vi "Punto 3.vi"() -> ()   [LabVIEW 2020]
panel:
  in  "Stop buttom":bool
  out "Value of destiny scale":dbl
  in  "Value of original scale":dbl
  in  "Operate":bool
  in  "Destiny scale":string(combo)
  in  "Original scale":string(combo)
  # "This program was created by Juan Bermúdez from the Army Aviation School\nat the Aircraft Engineering of the assignature of Programation II"
  # "How to use the software?:\n1- First, select the scale of longitude original.\n2- Second, select the new scale of longitude.\n3- Third, write the value of the longitude.\n4- Forth, push the buttom called = ''Operate''.\n5- Fifth, if you want to stop the software, push the buttom called = ''Stop buttom''.\n Enjoy the software :)"
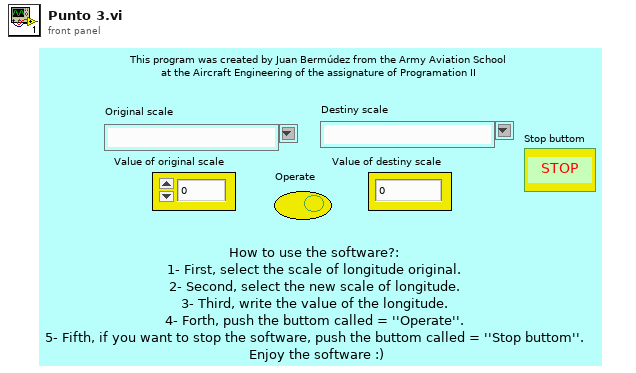
[diagram p1: front panel]
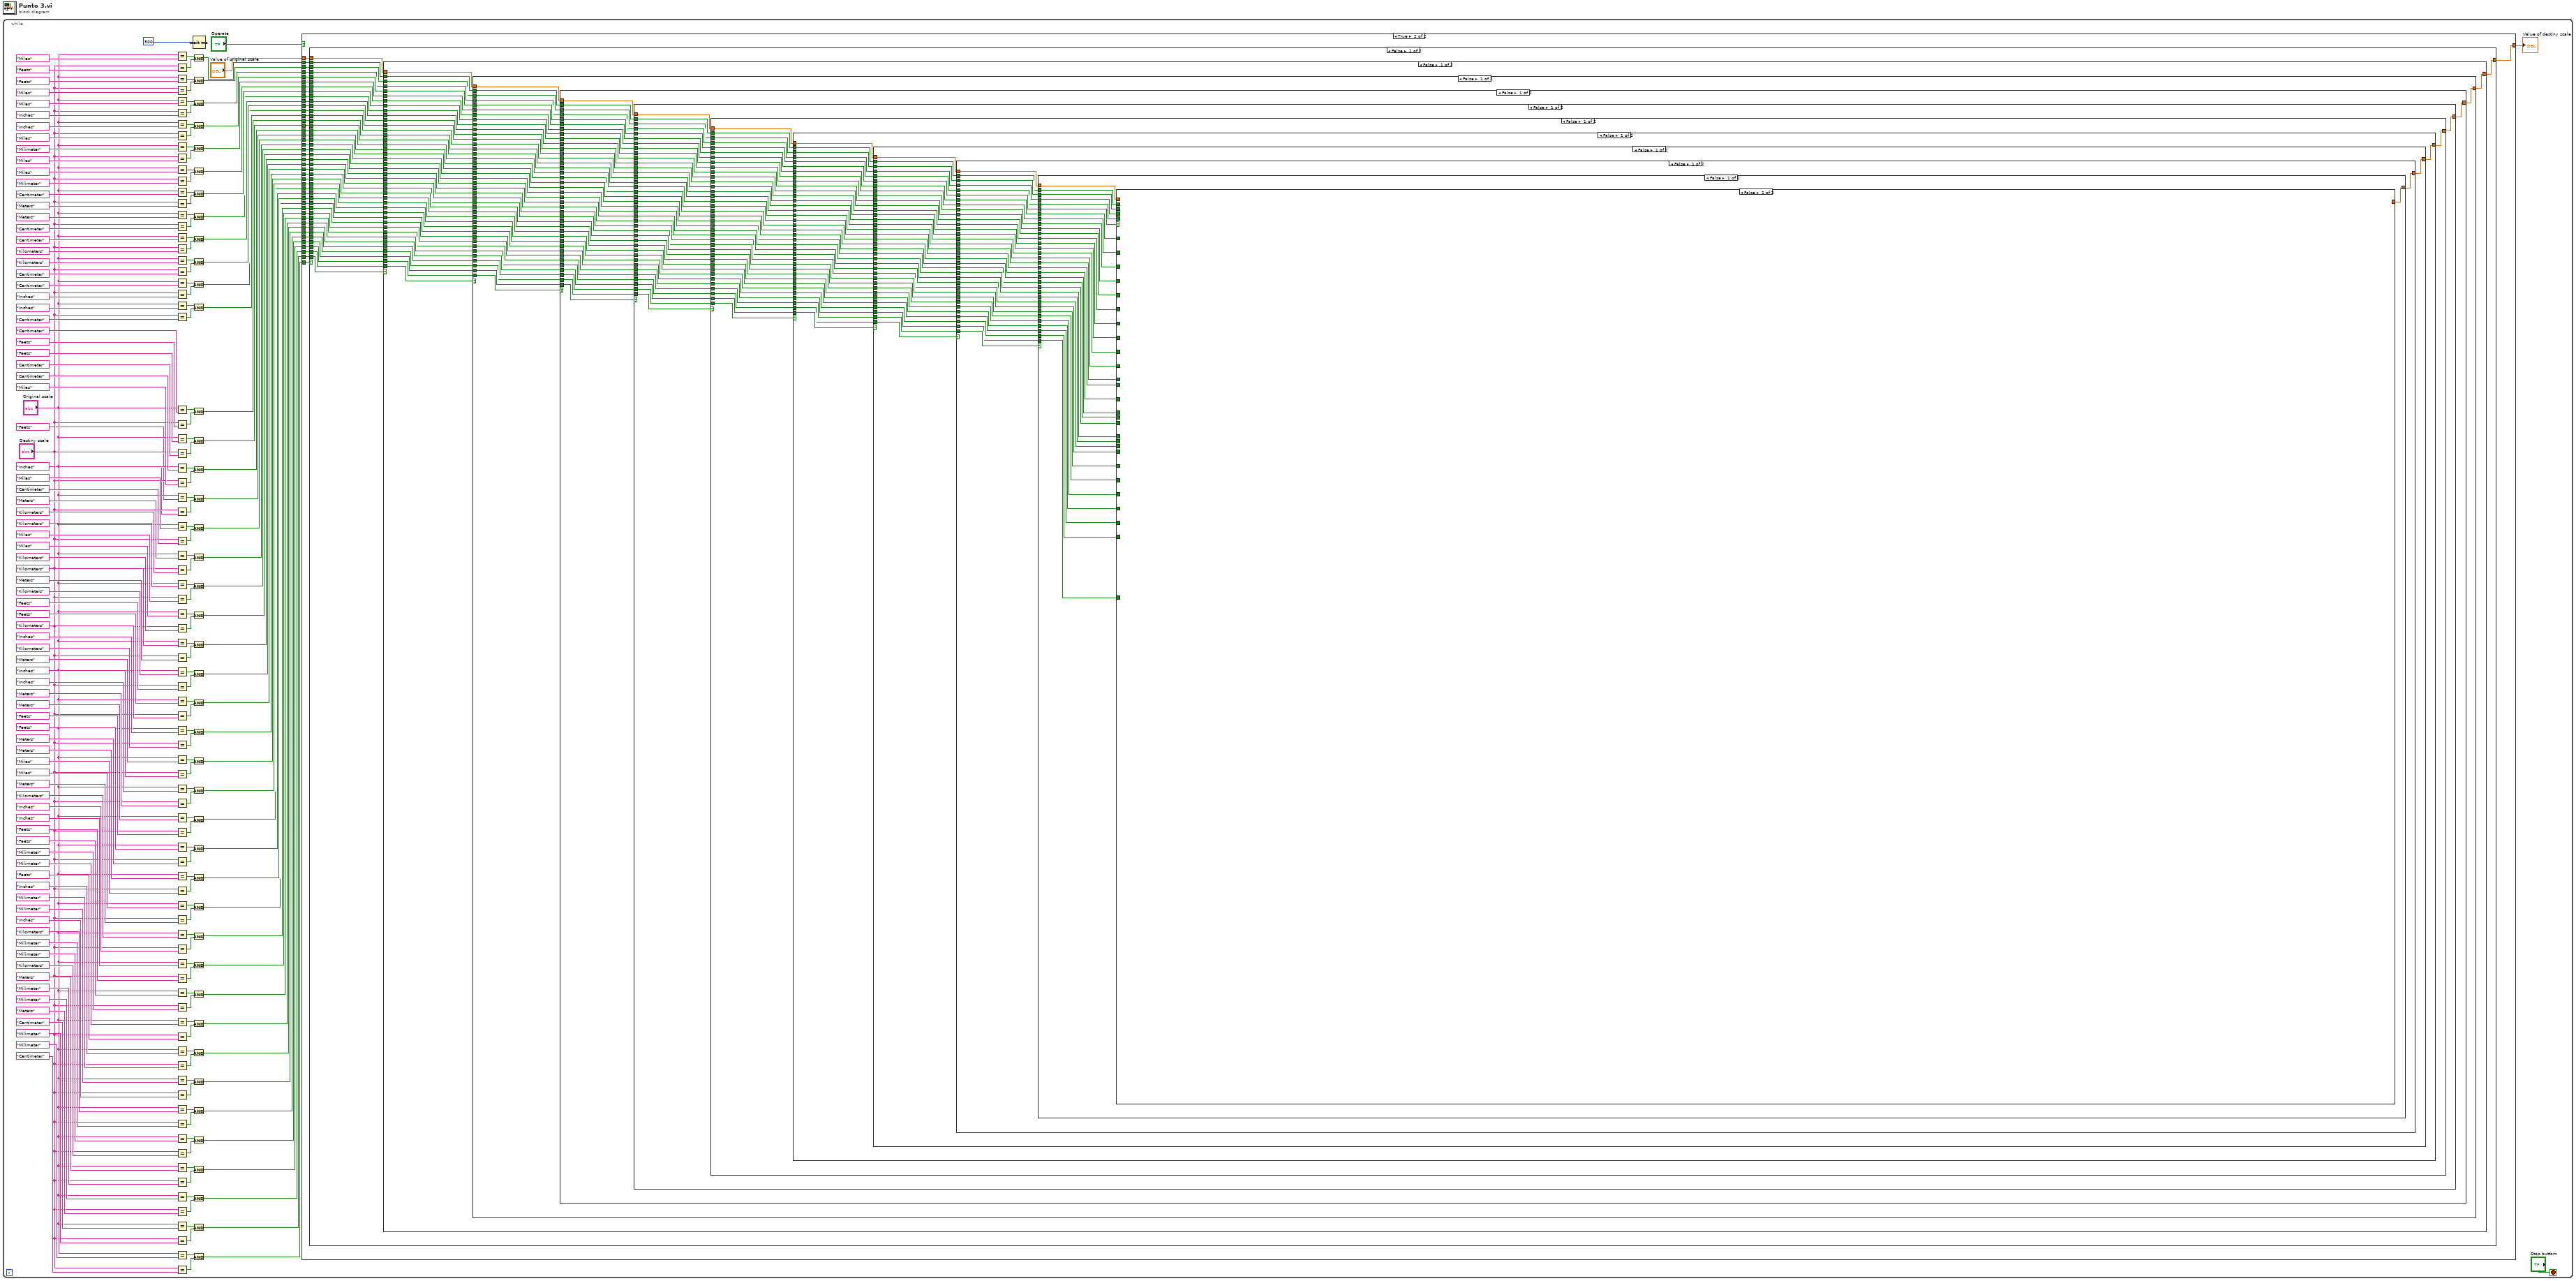
[diagram p0: block diagram]
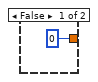
[diagram p2: hidden frame]
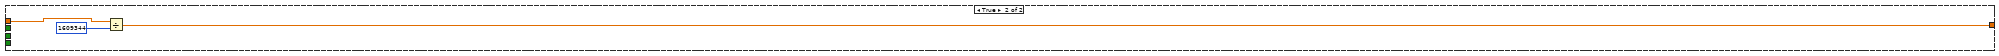
[diagram p3: hidden frame]
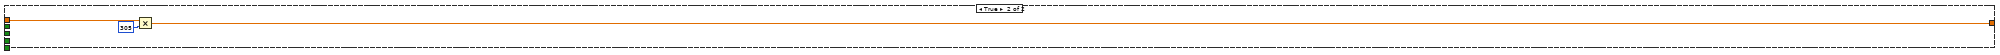
[diagram p4: hidden frame]
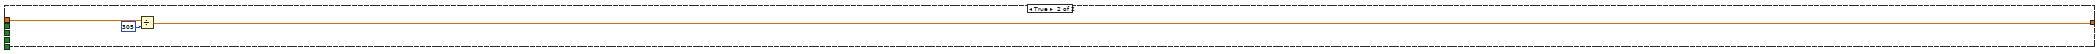
[diagram p5: hidden frame]
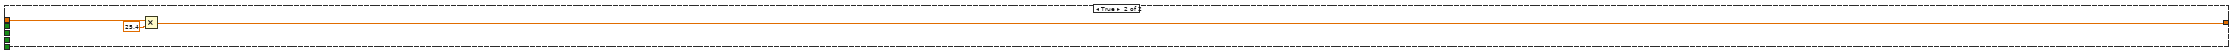
[diagram p6: hidden frame]
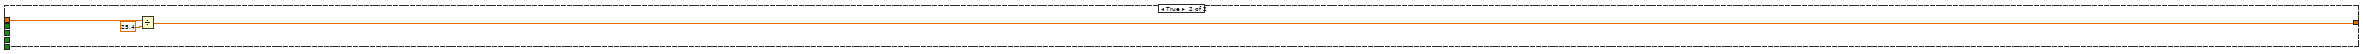
[diagram p7: hidden frame]
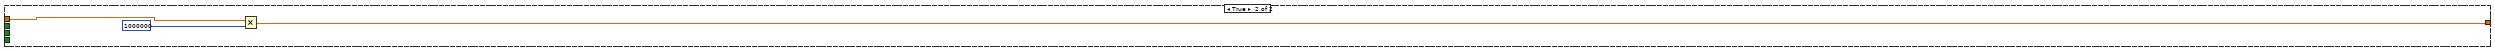
[diagram p8: hidden frame]
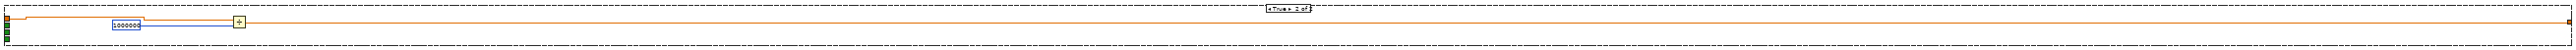
[diagram p9: hidden frame]
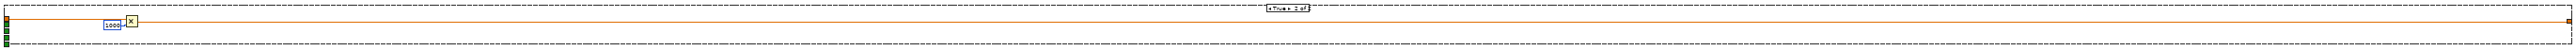
[diagram p10: hidden frame]
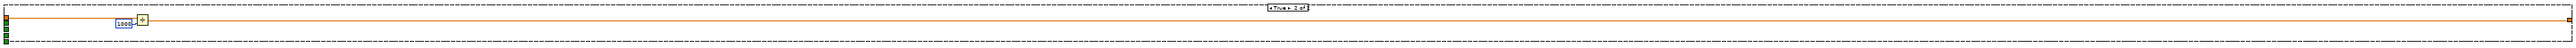
[diagram p11: hidden frame]
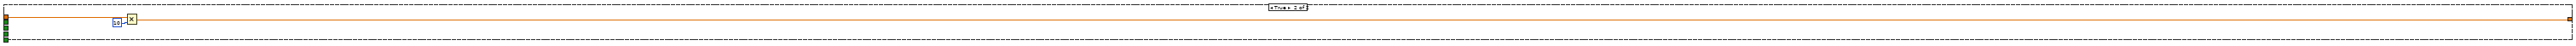
[diagram p12: hidden frame]
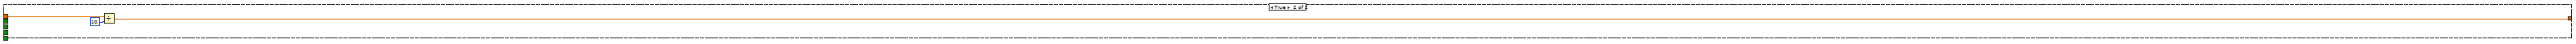
[diagram p13: hidden frame]
diagram:
  n1 = while {
    stop <- "Stop buttom" stop-if-true
    n2 = Equal?(x="Original scale", y="Miles") -> (x = y?=w10:bool)
    n3 = Equal?(x="Destiny scale", y="Feets") -> (x = y?=w11:bool)
    n4 = Equal?(x="Original scale", y="Feets") -> (x = y?=w16:bool)
    n5 = Equal?(x="Destiny scale", y="Miles") -> (x = y?=w15:bool)
    n6 = Equal?(x="Original scale", y="Miles") -> (x = y?=w20:bool)
    n7 = Equal?(x="Destiny scale", y="Inches") -> (x = y?=w21:bool)
    n8 = Equal?(x="Original scale", y="Inches") -> (x = y?=w26:bool)
    n9 = Equal?(x="Destiny scale", y="Miles") -> (x = y?=w25:bool)
    n10 = Equal?(x="Original scale", y="Milimeter") -> (x = y?=w163:bool)
    n11 = Equal?(x="Destiny scale", y="Miles") -> (x = y?=w164:bool)
    n12 = Equal?(x="Original scale", y="Miles") -> (x = y?=w159:bool)
    n13 = Equal?(x="Destiny scale", y="Milimeter") -> (x = y?=w158:bool)
    n14 = Equal?(x="Original scale", y="Centimeter") -> (x = y?=w153:bool)
    n15 = Equal?(x="Destiny scale", y="Meters") -> (x = y?=w154:bool)
    n16 = Equal?(x="Original scale", y="Meters") -> (x = y?=w148:bool)
    n17 = Equal?(x="Destiny scale", y="Centimeter") -> (x = y?=w149:bool)
    n18 = Equal?(x="Original scale", y="Centimeter") -> (x = y?=w143:bool)
    n19 = Equal?(x="Destiny scale", y="Kilometers") -> (x = y?=w144:bool)
    n20 = Equal?(x="Original scale", y="Kilometers") -> (x = y?=w139:bool)
    n21 = Equal?(x="Destiny scale", y="Centimeter") -> (x = y?=w138:bool)
    n22 = Equal?(x="Original scale", y="Centimeter") -> (x = y?=w133:bool)
    n23 = Equal?(x="Destiny scale", y="Inches") -> (x = y?=w134:bool)
    n24 = Equal?(x="Original scale", y="Inches") -> (x = y?=w128:bool)
    n25 = Equal?(x="Destiny scale", y="Centimeter") -> (x = y?=w129:bool)
    n26 = Equal?(x="Original scale", y="Centimeter") -> (x = y?=w123:bool)
    n27 = Equal?(x="Destiny scale", y="Feets") -> (x = y?=w124:bool)
    n28 = Equal?(x="Original scale", y="Feets") -> (x = y?=w118:bool)
    n29 = Equal?(x="Destiny scale", y="Centimeter") -> (x = y?=w119:bool)
    n30 = Equal?(x="Original scale", y="Centimeter") -> (x = y?=w114:bool)
    n31 = Equal?(x="Destiny scale", y="Miles") -> (x = y?=w113:bool)
    n32 = Equal?(x="Original scale", y="Feets") -> (x = y?=w32:bool)
    n33 = Equal?(x="Destiny scale", y="Inches") -> (x = y?=w31:bool)
    n34 = Equal?(x="Original scale", y="Miles") -> (x = y?=w108:bool)
    n35 = Equal?(x="Destiny scale", y="Centimeter") -> (x = y?=w109:bool)
    n36 = Equal?(x="Original scale", y="Meters") -> (x = y?=w103:bool)
    n37 = Equal?(x="Destiny scale", y="Kilometers") -> (x = y?=w104:bool)
    n38 = Equal?(x="Original scale", y="Kilometers") -> (x = y?=w41:bool)
    n39 = Equal?(x="Destiny scale", y="Miles") -> (x = y?=w42:bool)
    n40 = Equal?(x="Original scale", y="Miles") -> (x = y?=w44:bool)
    n41 = Equal?(x="Destiny scale", y="Kilometers") -> (x = y?=w43:bool)
    n42 = Equal?(x="Original scale", y="Kilometers") -> (x = y?=w98:bool)
    n43 = Equal?(x="Destiny scale", y="Meters") -> (x = y?=w99:bool)
    n44 = Equal?(x="Original scale", y="Kilometers") -> (x = y?=w54:bool)
    n45 = Equal?(x="Destiny scale", y="Feets") -> (x = y?=w53:bool)
    n46 = Equal?(x="Original scale", y="Feets") -> (x = y?=w48:bool)
    n47 = Equal?(x="Destiny scale", y="Kilometers") -> (x = y?=w49:bool)
    n48 = Equal?(x="Original scale", y="Inches") -> (x = y?=w59:bool)
    n49 = Equal?(x="Destiny scale", y="Kilometers") -> (x = y?=w58:bool)
    n50 = Equal?(x="Original scale", y="Meters") -> (x = y?=w93:bool)
    n51 = Equal?(x="Destiny scale", y="Inches") -> (x = y?=w94:bool)
    n52 = Equal?(x="Original scale", y="Inches") -> (x = y?=w89:bool)
    n53 = Equal?(x="Destiny scale", y="Meters") -> (x = y?=w88:bool)
    n54 = Equal?(x="Original scale", y="Meters") -> (x = y?=w83:bool)
    n55 = Equal?(x="Destiny scale", y="Feets") -> (x = y?=w84:bool)
    n56 = Equal?(x="Original scale", y="Feets") -> (x = y?=w82:bool)
    n57 = Equal?(x="Destiny scale", y="Meters") -> (x = y?=w81:bool)
    n58 = Equal?(x="Original scale", y="Meters") -> (x = y?=w74:bool)
    n59 = Equal?(x="Destiny scale", y="Miles") -> (x = y?=w73:bool)
    n60 = Equal?(x="Original scale", y="Miles") -> (x = y?=w71:bool)
    n61 = Equal?(x="Destiny scale", y="Meters") -> (x = y?=w72:bool)
    n62 = Equal?(x="Original scale", y="Kilometers") -> (x = y?=w63:bool)
    n63 = Equal?(x="Destiny scale", y="Inches") -> (x = y?=w64:bool)
    n64 = Equal?(x="Original scale", y="Inches") -> (x = y?=w33:bool)
    n65 = Equal?(x="Destiny scale", y="Feets") -> (x = y?=w34:bool)
    n66 = Equal?(x="Original scale", y="Feets") -> (x = y?=w168:bool)
    n67 = Equal?(x="Destiny scale", y="Milimeter") -> (x = y?=w169:bool)
    n68 = Equal?(x="Original scale", y="Milimeter") -> (x = y?=w174:bool)
    n69 = Equal?(x="Destiny scale", y="Feets") -> (x = y?=w173:bool)
    n70 = Equal?(x="Original scale", y="Inches") -> (x = y?=w179:bool)
    n71 = Equal?(x="Destiny scale", y="Milimeter") -> (x = y?=w178:bool)
    n72 = Equal?(x="Original scale", y="Milimeter") -> (x = y?=w183:bool)
    n73 = Equal?(x="Destiny scale", y="Inches") -> (x = y?=w184:bool)
    n74 = Equal?(x="Original scale", y="Kilometers") -> (x = y?=w188:bool)
    n75 = Equal?(x="Destiny scale", y="Milimeter") -> (x = y?=w189:bool)
    n76 = Equal?(x="Original scale", y="Milimeter") -> (x = y?=w194:bool)
    n77 = Equal?(x="Destiny scale", y="Kilometers") -> (x = y?=w193:bool)
    n78 = Equal?(x="Original scale", y="Meters") -> (x = y?=w198:bool)
    n79 = Equal?(x="Destiny scale", y="Milimeter") -> (x = y?=w199:bool)
    n80 = Equal?(x="Original scale", y="Milimeter") -> (x = y?=w204:bool)
    n81 = Equal?(x="Destiny scale", y="Meters") -> (x = y?=w203:bool)
    n82 = Equal?(x="Original scale", y="Centimeter") -> (x = y?=w208:bool)
    n83 = Equal?(x="Destiny scale", y="Milimeter") -> (x = y?=w209:bool)
    n84 = Equal?(x="Original scale", y="Milimeter") -> (x = y?=w215:bool)
    n85 = Equal?(x="Destiny scale", y="Centimeter") -> (x = y?=w214:bool)
    n86 = And(x=w10, y=w11) -> (x .and. y?=w5:bool)
    n87 = And(x=w16, y=w15) -> (x .and. y?=w12:bool)
    n88 = And(x=w20, y=w21) -> (x .and. y?=w17:bool)
    n89 = And(x=w26, y=w25) -> (x .and. y?=w22:bool)
    n90 = And(x=w163, y=w164) -> (x .and. y?=w160:bool)
    n91 = And(x=w159, y=w158) -> (x .and. y?=w155:bool)
    n92 = And(x=w153, y=w154) -> (x .and. y?=w150:bool)
    n93 = And(x=w148, y=w149) -> (x .and. y?=w145:bool)
    n94 = And(x=w143, y=w144) -> (x .and. y?=w140:bool)
    n95 = And(x=w139, y=w138) -> (x .and. y?=w137:bool)
    n96 = And(x=w133, y=w134) -> (x .and. y?=w130:bool)
    n97 = And(x=w128, y=w129) -> (x .and. y?=w125:bool)
    n98 = And(x=w123, y=w124) -> (x .and. y?=w120:bool)
    n99 = And(x=w118, y=w119) -> (x .and. y?=w115:bool)
    n100 = And(x=w114, y=w113) -> (x .and. y?=w110:bool)
    n101 = And(x=w32, y=w31) -> (x .and. y?=w27:bool)
    n102 = And(x=w108, y=w109) -> (x .and. y?=w105:bool)
    n103 = And(x=w103, y=w104) -> (x .and. y?=w100:bool)
    n104 = And(x=w41, y=w42) -> (x .and. y?=w38:bool)
    n105 = And(x=w44, y=w43) -> (x .and. y?=w35:bool)
    n106 = And(x=w98, y=w99) -> (x .and. y?=w95:bool)
    n107 = And(x=w54, y=w53) -> (x .and. y?=w50:bool)
    n108 = And(x=w48, y=w49) -> (x .and. y?=w45:bool)
    n109 = And(x=w59, y=w58) -> (x .and. y?=w55:bool)
    n110 = And(x=w93, y=w94) -> (x .and. y?=w90:bool)
    n111 = And(x=w89, y=w88) -> (x .and. y?=w85:bool)
    n112 = And(x=w83, y=w84) -> (x .and. y?=w78:bool)
    n113 = And(x=w82, y=w81) -> (x .and. y?=w75:bool)
    n114 = And(x=w74, y=w73) -> (x .and. y?=w66:bool)
    n115 = And(x=w71, y=w72) -> (x .and. y?=w65:bool)
    n116 = And(x=w63, y=w64) -> (x .and. y?=w60:bool)
    n117 = And(x=w33, y=w34) -> (x .and. y?=w28:bool)
    n118 = And(x=w168, y=w169) -> (x .and. y?=w165:bool)
    n119 = And(x=w174, y=w173) -> (x .and. y?=w170:bool)
    n120 = And(x=w179, y=w178) -> (x .and. y?=w175:bool)
    n121 = And(x=w183, y=w184) -> (x .and. y?=w180:bool)
    n122 = And(x=w188, y=w189) -> (x .and. y?=w185:bool)
    n123 = And(x=w194, y=w193) -> (x .and. y?=w190:bool)
    n124 = And(x=w198, y=w199) -> (x .and. y?=w195:bool)
    n125 = And(x=w204, y=w203) -> (x .and. y?=w200:bool)
    n126 = And(x=w208, y=w209) -> (x .and. y?=w205:bool)
    n127 = And(x=w215, y=w214) -> (x .and. y?=w212:bool)
    n128 = Wait (ms)(milliseconds to wait=500) -> ()  [unwired: 1 out]
    n129 = case shown="True" "Operate" {
      tunnel: w212 -> [_ w262]
      tunnel: "Value of original scale" -> [_ w261]
      tunnel: [0 w260] -> w210
      tunnel: w205 -> [_ w259]
      tunnel: w200 -> [_ w258]
      tunnel: w195 -> [_ w257]
      tunnel: w190 -> [_ w256]
      tunnel: w185 -> [_ w255]
      tunnel: w180 -> [_ w254]
      tunnel: w175 -> [_ w253]
      tunnel: w170 -> [_ w252]
      tunnel: w165 -> [_ w251]
      tunnel: w160 -> [_ w250]
      tunnel: w155 -> [_ w249]
      tunnel: w150 -> [_ w248]
      tunnel: w145 -> [_ w247]
      tunnel: w140 -> [_ w246]
      tunnel: w137 -> [_ w245]
      tunnel: w130 -> [_ w244]
      tunnel: w125 -> [_ w243]
      tunnel: w120 -> [_ w242]
      tunnel: w115 -> [_ w241]
      tunnel: w110 -> [_ w240]
      tunnel: w105 -> [_ w239]
      tunnel: w100 -> [_ w238]
      tunnel: w95 -> [_ w237]
      tunnel: w90 -> [_ w236]
      tunnel: w85 -> [_ w235]
      tunnel: w78 -> [_ w234]
      tunnel: w75 -> [_ w233]
      tunnel: w66 -> [_ w232]
      tunnel: w65 -> [_ w231]
      tunnel: w60 -> [_ w230]
      tunnel: w55 -> [_ w229]
      tunnel: w50 -> [_ w228]
      tunnel: w45 -> [_ w227]
      tunnel: w38 -> [_ w226]
      tunnel: w35 -> [_ w225]
      tunnel: w28 -> [_ w224]
      tunnel: w27 -> [_ w223]
      tunnel: w22 -> [_ w222]
      tunnel: w17 -> [_ w221]
      tunnel: w12 -> [_ w220]
      tunnel: w5 -> [_ w219]
      frame False {
      }
      frame True {
        n130 = case shown="False" w262 {
          tunnel: w261 -> [w304 w1332]
          tunnel: [w303 w1330] -> w260
          tunnel: w259 -> [w305 _]
          tunnel: w258 -> [w302 _]
          tunnel: w257 -> [w301 _]
          tunnel: w256 -> [w300 _]
          tunnel: w255 -> [w299 _]
          tunnel: w254 -> [w298 _]
          tunnel: w253 -> [w297 _]
          tunnel: w252 -> [w296 _]
          tunnel: w251 -> [w295 _]
          tunnel: w250 -> [w294 _]
          tunnel: w249 -> [w293 _]
          tunnel: w248 -> [w292 _]
          tunnel: w247 -> [w291 _]
          tunnel: w246 -> [w290 _]
          tunnel: w245 -> [w289 _]
          tunnel: w244 -> [w288 _]
          tunnel: w243 -> [w287 _]
          tunnel: w242 -> [w286 _]
          tunnel: w241 -> [w285 _]
          tunnel: w240 -> [w284 _]
          tunnel: w239 -> [w283 _]
          tunnel: w238 -> [w282 _]
          tunnel: w237 -> [w281 _]
          tunnel: w236 -> [w280 _]
          tunnel: w235 -> [w279 _]
          tunnel: w234 -> [w278 _]
          tunnel: w233 -> [w277 _]
          tunnel: w232 -> [w276 _]
          tunnel: w231 -> [w275 _]
          tunnel: w230 -> [w274 _]
          tunnel: w229 -> [w273 _]
          tunnel: w228 -> [w272 _]
          tunnel: w227 -> [w271 _]
          tunnel: w226 -> [w270 _]
          tunnel: w225 -> [w269 _]
          tunnel: w224 -> [w268 _]
          tunnel: w223 -> [w267 _]
          tunnel: w222 -> [w266 _]
          tunnel: w221 -> [w265 _]
          tunnel: w220 -> [w264 _]
          tunnel: w219 -> [w263 _]
          frame False {
            n131 = case shown="False" w305 {
              tunnel: w304 -> [w346 w1329]
              tunnel: [w345 w1327] -> w303
              tunnel: w302 -> [w347 _]
              tunnel: w301 -> [w344 _]
              tunnel: w300 -> [w343 _]
              tunnel: w299 -> [w342 _]
              tunnel: w298 -> [w341 _]
              tunnel: w297 -> [w340 _]
              tunnel: w296 -> [w339 _]
              tunnel: w295 -> [w338 _]
              tunnel: w294 -> [w337 _]
              tunnel: w293 -> [w336 _]
              tunnel: w292 -> [w335 _]
              tunnel: w291 -> [w334 _]
              tunnel: w290 -> [w333 _]
              tunnel: w289 -> [w332 _]
              tunnel: w288 -> [w331 _]
              tunnel: w287 -> [w330 _]
              tunnel: w286 -> [w329 _]
              tunnel: w285 -> [w328 _]
              tunnel: w284 -> [w327 _]
              tunnel: w283 -> [w326 _]
              tunnel: w282 -> [w325 _]
              tunnel: w281 -> [w324 _]
              tunnel: w280 -> [w323 _]
              tunnel: w279 -> [w322 _]
              tunnel: w278 -> [w321 _]
              tunnel: w277 -> [w320 _]
              tunnel: w276 -> [w319 _]
              tunnel: w275 -> [w318 _]
              tunnel: w274 -> [w317 _]
              tunnel: w273 -> [w316 _]
              tunnel: w272 -> [w315 _]
              tunnel: w271 -> [w314 _]
              tunnel: w270 -> [w313 _]
              tunnel: w269 -> [w312 _]
              tunnel: w268 -> [w311 _]
              tunnel: w267 -> [w310 _]
              tunnel: w266 -> [w309 _]
              tunnel: w265 -> [w308 _]
              tunnel: w264 -> [w307 _]
              tunnel: w263 -> [w306 _]
              frame False {
                n132 = case shown="False" w347 {
                  tunnel: w346 -> [w387 w1326]
                  tunnel: [w386 w1324] -> w345
                  tunnel: w344 -> [w388 _]
                  tunnel: w343 -> [w385 _]
                  tunnel: w342 -> [w384 _]
                  tunnel: w341 -> [w383 _]
                  tunnel: w340 -> [w382 _]
                  tunnel: w339 -> [w381 _]
                  tunnel: w338 -> [w380 _]
                  tunnel: w337 -> [w379 _]
                  tunnel: w336 -> [w378 _]
                  tunnel: w335 -> [w377 _]
                  tunnel: w334 -> [w376 _]
                  tunnel: w333 -> [w375 _]
                  tunnel: w332 -> [w374 _]
                  tunnel: w331 -> [w373 _]
                  tunnel: w330 -> [w372 _]
                  tunnel: w329 -> [w371 _]
                  tunnel: w328 -> [w370 _]
                  tunnel: w327 -> [w369 _]
                  tunnel: w326 -> [w368 _]
                  tunnel: w325 -> [w367 _]
                  tunnel: w324 -> [w366 _]
                  tunnel: w323 -> [w365 _]
                  tunnel: w322 -> [w364 _]
                  tunnel: w321 -> [w363 _]
                  tunnel: w320 -> [w362 _]
                  tunnel: w319 -> [w361 _]
                  tunnel: w318 -> [w360 _]
                  tunnel: w317 -> [w359 _]
                  tunnel: w316 -> [w358 _]
                  tunnel: w315 -> [w357 _]
                  tunnel: w314 -> [w356 _]
                  tunnel: w313 -> [w355 _]
                  tunnel: w312 -> [w354 _]
                  tunnel: w311 -> [w353 _]
                  tunnel: w310 -> [w352 _]
                  tunnel: w309 -> [w351 _]
                  tunnel: w308 -> [w350 _]
                  tunnel: w307 -> [w349 _]
                  tunnel: w306 -> [w348 _]
                  frame False {
                    n133 = case shown="False" w388 {
                      tunnel: w387 -> [w427 w1323]
                      tunnel: [w426 w1321] -> w386
                      tunnel: w385 -> [w428 _]
                      tunnel: w384 -> [w425 _]
                      tunnel: w383 -> [w424 _]
                      tunnel: w382 -> [w423 _]
                      tunnel: w381 -> [w422 _]
                      tunnel: w380 -> [w421 _]
                      tunnel: w379 -> [w420 _]
                      tunnel: w378 -> [w419 _]
                      tunnel: w377 -> [w418 _]
                      tunnel: w376 -> [w417 _]
                      tunnel: w375 -> [w416 _]
                      tunnel: w374 -> [w415 _]
                      tunnel: w373 -> [w414 _]
                      tunnel: w372 -> [w413 _]
                      tunnel: w371 -> [w412 _]
                      tunnel: w370 -> [w411 _]
                      tunnel: w369 -> [w410 _]
                      tunnel: w368 -> [w409 _]
                      tunnel: w367 -> [w408 _]
                      tunnel: w366 -> [w407 _]
                      tunnel: w365 -> [w406 _]
                      tunnel: w364 -> [w405 _]
                      tunnel: w363 -> [w404 _]
                      tunnel: w362 -> [w403 _]
                      tunnel: w361 -> [w402 _]
                      tunnel: w360 -> [w401 _]
                      tunnel: w359 -> [w400 _]
                      tunnel: w358 -> [w399 _]
                      tunnel: w357 -> [w398 _]
                      tunnel: w356 -> [w397 _]
                      tunnel: w355 -> [w396 _]
                      tunnel: w354 -> [w395 _]
                      tunnel: w353 -> [w394 _]
                      tunnel: w352 -> [w393 _]
                      tunnel: w351 -> [w392 _]
                      tunnel: w350 -> [w391 _]
                      tunnel: w349 -> [w390 _]
                      tunnel: w348 -> [w389 _]
                      frame False {
                        n134 = case shown="False" w428 {
                          tunnel: w427 -> [w466 w1319]
                          tunnel: [w465 w1318] -> w426
                          tunnel: w425 -> [w467 _]
                          tunnel: w424 -> [w464 _]
                          tunnel: w423 -> [w463 _]
                          tunnel: w422 -> [w462 _]
                          tunnel: w421 -> [w461 _]
                          tunnel: w420 -> [w460 _]
                          tunnel: w419 -> [w459 _]
                          tunnel: w418 -> [w458 _]
                          tunnel: w417 -> [w457 _]
                          tunnel: w416 -> [w456 _]
                          tunnel: w415 -> [w455 _]
                          tunnel: w414 -> [w454 _]
                          tunnel: w413 -> [w453 _]
                          tunnel: w412 -> [w452 _]
                          tunnel: w411 -> [w451 _]
                          tunnel: w410 -> [w450 _]
                          tunnel: w409 -> [w449 _]
                          tunnel: w408 -> [w448 _]
                          tunnel: w407 -> [w447 _]
                          tunnel: w406 -> [w446 _]
                          tunnel: w405 -> [w445 _]
                          tunnel: w404 -> [w444 _]
                          tunnel: w403 -> [w443 _]
                          tunnel: w402 -> [w442 _]
                          tunnel: w401 -> [w441 _]
                          tunnel: w400 -> [w440 _]
                          tunnel: w399 -> [w439 _]
                          tunnel: w398 -> [w438 _]
                          tunnel: w397 -> [w437 _]
                          tunnel: w396 -> [w436 _]
                          tunnel: w395 -> [w435 _]
                          tunnel: w394 -> [w434 _]
                          tunnel: w393 -> [w433 _]
                          tunnel: w392 -> [w432 _]
                          tunnel: w391 -> [w431 _]
                          tunnel: w390 -> [w430 _]
                          tunnel: w389 -> [w429 _]
                          frame False {
                            n135 = case shown="False" w467 {
                              tunnel: w466 -> [w504 w1316]
                              tunnel: [w503 w1315] -> w465
                              tunnel: w464 -> [w505 _]
                              tunnel: w463 -> [w502 _]
                              tunnel: w462 -> [w501 _]
                              tunnel: w461 -> [w500 _]
                              tunnel: w460 -> [w499 _]
                              tunnel: w459 -> [w498 _]
                              tunnel: w458 -> [w497 _]
                              tunnel: w457 -> [w496 _]
                              tunnel: w456 -> [w495 _]
                              tunnel: w455 -> [w494 _]
                              tunnel: w454 -> [w493 _]
                              tunnel: w453 -> [w492 _]
                              tunnel: w452 -> [w491 _]
                              tunnel: w451 -> [w490 _]
                              tunnel: w450 -> [w489 _]
                              tunnel: w449 -> [w488 _]
                              tunnel: w448 -> [w487 _]
                              tunnel: w447 -> [w486 _]
                              tunnel: w446 -> [w485 _]
                              tunnel: w445 -> [w484 _]
                              tunnel: w444 -> [w483 _]
                              tunnel: w443 -> [w482 _]
                              tunnel: w442 -> [w481 _]
                              tunnel: w441 -> [w480 _]
                              tunnel: w440 -> [w479 _]
                              tunnel: w439 -> [w478 _]
                              tunnel: w438 -> [w477 _]
                              tunnel: w437 -> [w476 _]
                              tunnel: w436 -> [w475 _]
                              tunnel: w435 -> [w474 _]
                              tunnel: w434 -> [w473 _]
                              tunnel: w433 -> [w472 _]
                              tunnel: w432 -> [w471 _]
                              tunnel: w431 -> [w470 _]
                              tunnel: w430 -> [w469 _]
                              tunnel: w429 -> [w468 _]
                              frame False {
                                n136 = case shown="False" w505 {
                                tunnel: w504 -> [w541 w1314]
                                tunnel: [w540 w1312] -> w503
                                tunnel: w502 -> [w542 _]
                                tunnel: w501 -> [w539 _]
                                tunnel: w500 -> [w538 _]
                                tunnel: w499 -> [w537 _]
                                tunnel: w498 -> [w536 _]
                                tunnel: w497 -> [w535 _]
                                tunnel: w496 -> [w534 _]
                                tunnel: w495 -> [w533 _]
                                tunnel: w494 -> [w532 _]
                                tunnel: w493 -> [w531 _]
                                tunnel: w492 -> [w530 _]
                                tunnel: w491 -> [w529 _]
                                tunnel: w490 -> [w528 _]
                                tunnel: w489 -> [w527 _]
                                tunnel: w488 -> [w526 _]
                                tunnel: w487 -> [w525 _]
                                tunnel: w486 -> [w524 _]
                                tunnel: w485 -> [w523 _]
                                tunnel: w484 -> [w522 _]
                                tunnel: w483 -> [w521 _]
                                tunnel: w482 -> [w520 _]
                                tunnel: w481 -> [w519 _]
                                tunnel: w480 -> [w518 _]
                                tunnel: w479 -> [w517 _]
                                tunnel: w478 -> [w516 _]
                                tunnel: w477 -> [w515 _]
                                tunnel: w476 -> [w514 _]
                                tunnel: w475 -> [w513 _]
                                tunnel: w474 -> [w512 _]
                                tunnel: w473 -> [w511 _]
                                tunnel: w472 -> [w510 _]
                                tunnel: w471 -> [w509 _]
                                tunnel: w470 -> [w508 _]
                                tunnel: w469 -> [w507 _]
                                tunnel: w468 -> [w506 _]
                                frame False {
                                n137 = case shown="False" w542 {
                                tunnel: w541 -> [w577 w1311]
                                tunnel: [w576 w1309] -> w540
                                tunnel: w539 -> [w578 _]
                                tunnel: w538 -> [w575 _]
                                tunnel: w537 -> [w574 _]
                                tunnel: w536 -> [w573 _]
                                tunnel: w535 -> [w572 _]
                                tunnel: w534 -> [w571 _]
                                tunnel: w533 -> [w570 _]
                                tunnel: w532 -> [w569 _]
                                tunnel: w531 -> [w568 _]
                                tunnel: w530 -> [w567 _]
                                tunnel: w529 -> [w566 _]
                                tunnel: w528 -> [w565 _]
                                tunnel: w527 -> [w564 _]
                                tunnel: w526 -> [w563 _]
                                tunnel: w525 -> [w562 _]
                                tunnel: w524 -> [w561 _]
                                tunnel: w523 -> [w560 _]
                                tunnel: w522 -> [w559 _]
                                tunnel: w521 -> [w558 _]
                                tunnel: w520 -> [w557 _]
                                tunnel: w519 -> [w556 _]
                                tunnel: w518 -> [w555 _]
                                tunnel: w517 -> [w554 _]
                                tunnel: w516 -> [w553 _]
                                tunnel: w515 -> [w552 _]
                                tunnel: w514 -> [w551 _]
                                tunnel: w513 -> [w550 _]
                                tunnel: w512 -> [w549 _]
                                tunnel: w511 -> [w548 _]
                                tunnel: w510 -> [w547 _]
                                tunnel: w509 -> [w546 _]
                                tunnel: w508 -> [w545 _]
                                tunnel: w507 -> [w544 _]
                                tunnel: w506 -> [w543 _]
                                frame False {
                                n138 = case shown="False" w578 {
                                tunnel: w577 -> [w612 w1307]
                                tunnel: [w611 w1306] -> w576
                                tunnel: w575 -> [w613 _]
                                tunnel: w574 -> [w610 _]
                                tunnel: w573 -> [w609 _]
                                tunnel: w572 -> [w608 _]
                                tunnel: w571 -> [w607 _]
                                tunnel: w570 -> [w606 _]
                                tunnel: w569 -> [w605 _]
                                tunnel: w568 -> [w604 _]
                                tunnel: w567 -> [w603 _]
                                tunnel: w566 -> [w602 _]
                                tunnel: w565 -> [w601 _]
                                tunnel: w564 -> [w600 _]
                                tunnel: w563 -> [w599 _]
                                tunnel: w562 -> [w598 _]
                                tunnel: w561 -> [w597 _]
                                tunnel: w560 -> [w596 _]
                                tunnel: w559 -> [w595 _]
                                tunnel: w558 -> [w594 _]
                                tunnel: w557 -> [w593 _]
                                tunnel: w556 -> [w592 _]
                                tunnel: w555 -> [w591 _]
                                tunnel: w554 -> [w590 _]
                                tunnel: w553 -> [w589 _]
                                tunnel: w552 -> [w588 _]
                                tunnel: w551 -> [w587 _]
                                tunnel: w550 -> [w586 _]
                                tunnel: w549 -> [w585 _]
                                tunnel: w548 -> [w584 _]
                                tunnel: w547 -> [w583 _]
                                tunnel: w546 -> [w582 _]
                                tunnel: w545 -> [w581 _]
                                tunnel: w544 -> [w580 _]
                                tunnel: w543 -> [w579 _]
                                frame False {
                                n139 = case shown="False" w613 {
                                tunnel: w612 -> [w647 w1305]
                                tunnel: [w645 w1303] -> w611
                                tunnel: w610 -> [w646 _]
                                tunnel: w609 -> [w644 _]
                                tunnel: w608 -> [w643 _]
                                tunnel: w607 -> [w642 _]
                                tunnel: w606 -> [w641 _]
                                tunnel: w605 -> [w640 _]
                                tunnel: w604 -> [w639 _]
                                tunnel: w603 -> [w638 _]
                                tunnel: w602 -> [w637 _]
                                tunnel: w601 -> [w636 _]
                                tunnel: w600 -> [w635 _]
                                tunnel: w599 -> [w634 _]
                                tunnel: w598 -> [w633 _]
                                tunnel: w597 -> [w632 _]
                                tunnel: w596 -> [w631 _]
                                tunnel: w595 -> [w630 _]
                                tunnel: w594 -> [w629 _]
                                tunnel: w593 -> [w628 _]
                                tunnel: w592 -> [w627 _]
                                tunnel: w591 -> [w626 _]
                                tunnel: w590 -> [w625 _]
                                tunnel: w589 -> [w624 _]
                                tunnel: w588 -> [w623 _]
                                tunnel: w587 -> [w622 _]
                                tunnel: w586 -> [w621 _]
                                tunnel: w585 -> [w620 _]
                                tunnel: w584 -> [w619 _]
                                tunnel: w583 -> [w618 _]
                                tunnel: w582 -> [w617 _]
                                tunnel: w581 -> [w616 _]
                                tunnel: w580 -> [w615 _]
                                tunnel: w579 -> [w614 _]
                                frame False {
                                n140 = case shown="False" w646 {
                                tunnel: w647 -> [w680 w1301]
                                tunnel: [w679 w1300] -> w645
                                tunnel: w644 -> [w678 _]
                                tunnel: w643 -> [w677 _]
                                tunnel: w642 -> [w676 _]
                                tunnel: w641 -> [w675 _]
                                tunnel: w640 -> [w674 _]
                                tunnel: w639 -> [w673 _]
                                tunnel: w638 -> [w672 _]
                                tunnel: w637 -> [w671 _]
                                tunnel: w636 -> [w670 _]
                                tunnel: w635 -> [w669 _]
                                tunnel: w634 -> [w668 _]
                                tunnel: w633 -> [w667 _]
                                tunnel: w632 -> [w666 _]
                                tunnel: w631 -> [w665 _]
                                tunnel: w630 -> [w664 _]
                                tunnel: w629 -> [w663 _]
                                tunnel: w628 -> [w662 _]
                                tunnel: w627 -> [w661 _]
                                tunnel: w626 -> [w660 _]
                                tunnel: w625 -> [w659 _]
                                tunnel: w624 -> [w658 _]
                                tunnel: w623 -> [w657 _]
                                tunnel: w622 -> [w656 _]
                                tunnel: w621 -> [w655 _]
                                tunnel: w620 -> [w654 _]
                                tunnel: w619 -> [w653 _]
                                tunnel: w618 -> [w652 _]
                                tunnel: w617 -> [w651 _]
                                tunnel: w616 -> [w650 _]
                                tunnel: w615 -> [w649 _]
                                tunnel: w614 -> [w648 _]
                                frame False {
                                n141 = case shown="False" w678 {
                                tunnel: w680 -> [w711 w1298]
                                tunnel: [w710 w1297] -> w679
                                tunnel: w677 -> [w712 _]
                                tunnel: w676 -> [w709 _]
                                tunnel: w675 -> [w708 _]
                                tunnel: w674 -> [w707 _]
                                tunnel: w673 -> [w706 _]
                                tunnel: w672 -> [w705 _]
                                tunnel: w671 -> [w704 _]
                                tunnel: w670 -> [w703 _]
                                tunnel: w669 -> [w702 _]
                                tunnel: w668 -> [w701 _]
                                tunnel: w667 -> [w700 _]
                                tunnel: w666 -> [w699 _]
                                tunnel: w665 -> [w698 _]
                                tunnel: w664 -> [w697 _]
                                tunnel: w663 -> [w696 _]
                                tunnel: w662 -> [w695 _]
                                tunnel: w661 -> [w694 _]
                                tunnel: w660 -> [w693 _]
                                tunnel: w659 -> [w692 _]
                                tunnel: w658 -> [w691 _]
                                tunnel: w657 -> [w690 _]
                                tunnel: w656 -> [w689 _]
                                tunnel: w655 -> [w688 _]
                                tunnel: w654 -> [w687 _]
                                tunnel: w653 -> [w686 _]
                                tunnel: w652 -> [w685 _]
                                tunnel: w651 -> [w684 _]
                                tunnel: w650 -> [w683 _]
                                tunnel: w649 -> [w682 _]
                                tunnel: w648 -> [w681 _]
                                frame False {
                                n142 = case shown="False" w712 {
                                tunnel: w711 -> [w742 w1295]
                                tunnel: [w741 w1294] -> w710
                                tunnel: w709 -> [w743 _]
                                tunnel: w708 -> [w740 _]
                                tunnel: w707 -> [w739 _]
                                tunnel: w706 -> [w738 _]
                                tunnel: w705 -> [w737 _]
                                tunnel: w704 -> [w736 _]
                                tunnel: w703 -> [w735 _]
                                tunnel: w702 -> [w734 _]
                                tunnel: w701 -> [w733 _]
                                tunnel: w700 -> [w732 _]
                                tunnel: w699 -> [w731 _]
                                tunnel: w698 -> [w730 _]
                                tunnel: w697 -> [w729 _]
                                tunnel: w696 -> [w728 _]
                                tunnel: w695 -> [w727 _]
                                tunnel: w694 -> [w726 _]
                                tunnel: w693 -> [w725 _]
                                tunnel: w692 -> [w724 _]
                                tunnel: w691 -> [w723 _]
                                tunnel: w690 -> [w722 _]
                                tunnel: w689 -> [w721 _]
                                tunnel: w688 -> [w720 _]
                                tunnel: w687 -> [w719 _]
                                tunnel: w686 -> [w718 _]
                                tunnel: w685 -> [w717 _]
                                tunnel: w684 -> [w716 _]
                                tunnel: w683 -> [w715 _]
                                tunnel: w682 -> [w714 _]
                                tunnel: w681 -> [w713 _]
                                frame False {
                                n143 = case shown="False" w743 {
                                tunnel: w742 -> [w772 w1293]
                                tunnel: [w771 w1291] -> w741
                                tunnel: w740 -> [w773 _]
                                tunnel: w739 -> [w770 _]
                                tunnel: w738 -> [w769 _]
                                tunnel: w737 -> [w768 _]
                                tunnel: w736 -> [w767 _]
                                tunnel: w735 -> [w766 _]
                                tunnel: w734 -> [w765 _]
                                tunnel: w733 -> [w764 _]
                                tunnel: w732 -> [w763 _]
                                tunnel: w731 -> [w762 _]
                                tunnel: w730 -> [w761 _]
                                tunnel: w729 -> [w760 _]
                                tunnel: w728 -> [w759 _]
                                tunnel: w727 -> [w758 _]
                                tunnel: w726 -> [w757 _]
                                tunnel: w725 -> [w756 _]
                                tunnel: w724 -> [w755 _]
                                tunnel: w723 -> [w754 _]
                                tunnel: w722 -> [w753 _]
                                tunnel: w721 -> [w752 _]
                                tunnel: w720 -> [w751 _]
                                tunnel: w719 -> [w750 _]
                                tunnel: w718 -> [w749 _]
                                tunnel: w717 -> [w748 _]
                                tunnel: w716 -> [w747 _]
                                tunnel: w715 -> [w746 _]
                                tunnel: w714 -> [w745 _]
                                tunnel: w713 -> [w744 _]
                                frame False {
                                n144 = case shown="False" w773 {
                                tunnel: w772 -> [w801 w1289]
                                tunnel: [w800 w1288] -> w771
                                tunnel: w770 -> [w802 _]
                                tunnel: w769 -> [w799 _]
                                tunnel: w768 -> [w798 _]
                                tunnel: w767 -> [w797 _]
                                tunnel: w766 -> [w796 _]
                                tunnel: w765 -> [w795 _]
                                tunnel: w764 -> [w794 _]
                                tunnel: w763 -> [w793 _]
                                tunnel: w762 -> [w792 _]
                                tunnel: w761 -> [w791 _]
                                tunnel: w760 -> [w790 _]
                                tunnel: w759 -> [w789 _]
                                tunnel: w758 -> [w788 _]
                                tunnel: w757 -> [w787 _]
                                tunnel: w756 -> [w786 _]
                                tunnel: w755 -> [w785 _]
                                tunnel: w754 -> [w784 _]
                                tunnel: w753 -> [w783 _]
                                tunnel: w752 -> [w782 _]
                                tunnel: w751 -> [w781 _]
                                tunnel: w750 -> [w780 _]
                                tunnel: w749 -> [w779 _]
                                tunnel: w748 -> [w778 _]
                                tunnel: w747 -> [w777 _]
                                tunnel: w746 -> [w776 _]
                                tunnel: w745 -> [w775 _]
                                tunnel: w744 -> [w774 _]
                                frame False {
                                n145 = case shown="False" w802 {
                                tunnel: w801 -> [w829 w1287]
                                tunnel: [w828 w1285] -> w800
                                tunnel: w799 -> [w830 _]
                                tunnel: w798 -> [w827 _]
                                tunnel: w797 -> [w826 _]
                                tunnel: w796 -> [w825 _]
                                tunnel: w795 -> [w824 _]
                                tunnel: w794 -> [w823 _]
                                tunnel: w793 -> [w822 _]
                                tunnel: w792 -> [w821 _]
                                tunnel: w791 -> [w820 _]
                                tunnel: w790 -> [w819 _]
                                tunnel: w789 -> [w818 _]
                                tunnel: w788 -> [w817 _]
                                tunnel: w787 -> [w816 _]
                                tunnel: w786 -> [w815 _]
                                tunnel: w785 -> [w814 _]
                                tunnel: w784 -> [w813 _]
                                tunnel: w783 -> [w812 _]
                                tunnel: w782 -> [w811 _]
                                tunnel: w781 -> [w810 _]
                                tunnel: w780 -> [w809 _]
                                tunnel: w779 -> [w808 _]
                                tunnel: w778 -> [w807 _]
                                tunnel: w777 -> [w806 _]
                                tunnel: w776 -> [w805 _]
                                tunnel: w775 -> [w804 _]
                                tunnel: w774 -> [w803 _]
                                frame False {
                                n146 = case shown="False" w830 {
                                tunnel: w829 -> [w856 w1283]
                                tunnel: [w855 w1282] -> w828
                                tunnel: w827 -> [w857 _]
                                tunnel: w826 -> [w854 _]
                                tunnel: w825 -> [w853 _]
                                tunnel: w824 -> [w852 _]
                                tunnel: w823 -> [w851 _]
                                tunnel: w822 -> [w850 _]
                                tunnel: w821 -> [w849 _]
                                tunnel: w820 -> [w848 _]
                                tunnel: w819 -> [w847 _]
                                tunnel: w818 -> [w846 _]
                                tunnel: w817 -> [w845 _]
                                tunnel: w816 -> [w844 _]
                                tunnel: w815 -> [w843 _]
                                tunnel: w814 -> [w842 _]
                                tunnel: w813 -> [w841 _]
                                tunnel: w812 -> [w840 _]
                                tunnel: w811 -> [w839 _]
                                tunnel: w810 -> [w838 _]
                                tunnel: w809 -> [w837 _]
                                tunnel: w808 -> [w836 _]
                                tunnel: w807 -> [w835 _]
                                tunnel: w806 -> [w834 _]
                                tunnel: w805 -> [w833 _]
                                tunnel: w804 -> [w832 _]
                                tunnel: w803 -> [w831 _]
                                frame False {
                                n147 = case shown="False" w857 {
                                tunnel: w856 -> [w882 w1281]
                                tunnel: [w881 w1279] -> w855
                                tunnel: w854 -> [w883 _]
                                tunnel: w853 -> [w880 _]
                                tunnel: w852 -> [w879 _]
                                tunnel: w851 -> [w878 _]
                                tunnel: w850 -> [w877 _]
                                tunnel: w849 -> [w876 _]
                                tunnel: w848 -> [w875 _]
                                tunnel: w847 -> [w874 _]
                                tunnel: w846 -> [w873 _]
                                tunnel: w845 -> [w872 _]
                                tunnel: w844 -> [w871 _]
                                tunnel: w843 -> [w870 _]
                                tunnel: w842 -> [w869 _]
                                tunnel: w841 -> [w868 _]
                                tunnel: w840 -> [w867 _]
                                tunnel: w839 -> [w866 _]
                                tunnel: w838 -> [w865 _]
                                tunnel: w837 -> [w864 _]
                                tunnel: w836 -> [w863 _]
                                tunnel: w835 -> [w862 _]
                                tunnel: w834 -> [w861 _]
                                tunnel: w833 -> [w860 _]
                                tunnel: w832 -> [w859 _]
                                tunnel: w831 -> [w858 _]
                                frame False {
                                n148 = case shown="False" w883 {
                                tunnel: w882 -> [w907 w1277]
                                tunnel: [w906 w1276] -> w881
                                tunnel: w880 -> [w908 _]
                                tunnel: w879 -> [w905 _]
                                tunnel: w878 -> [w904 _]
                                tunnel: w877 -> [w903 _]
                                tunnel: w876 -> [w902 _]
                                tunnel: w875 -> [w901 _]
                                tunnel: w874 -> [w900 _]
                                tunnel: w873 -> [w899 _]
                                tunnel: w872 -> [w898 _]
                                tunnel: w871 -> [w897 _]
                                tunnel: w870 -> [w896 _]
                                tunnel: w869 -> [w895 _]
                                tunnel: w868 -> [w894 _]
                                tunnel: w867 -> [w893 _]
                                tunnel: w866 -> [w892 _]
                                tunnel: w865 -> [w891 _]
                                tunnel: w864 -> [w890 _]
                                tunnel: w863 -> [w889 _]
                                tunnel: w862 -> [w888 _]
                                tunnel: w861 -> [w887 _]
                                tunnel: w860 -> [w886 _]
                                tunnel: w859 -> [w885 _]
                                tunnel: w858 -> [w884 _]
                                frame False {
                                n149 = case shown="False" w908 {
                                tunnel: w907 -> [w931 w1275]
                                tunnel: [w930 w1273] -> w906
                                tunnel: w905 -> [w932 _]
                                tunnel: w904 -> [w929 _]
                                tunnel: w903 -> [w928 _]
                                tunnel: w902 -> [w927 _]
                                tunnel: w901 -> [w926 _]
                                tunnel: w900 -> [w925 _]
                                tunnel: w899 -> [w924 _]
                                tunnel: w898 -> [w923 _]
                                tunnel: w897 -> [w922 _]
                                tunnel: w896 -> [w921 _]
                                tunnel: w895 -> [w920 _]
                                tunnel: w894 -> [w919 _]
                                tunnel: w893 -> [w918 _]
                                tunnel: w892 -> [w917 _]
                                tunnel: w891 -> [w916 _]
                                tunnel: w890 -> [w915 _]
                                tunnel: w889 -> [w914 _]
                                tunnel: w888 -> [w913 _]
                                tunnel: w887 -> [w912 _]
                                tunnel: w886 -> [w911 _]
                                tunnel: w885 -> [w910 _]
                                tunnel: w884 -> [w909 _]
                                frame False {
                                n150 = case shown="False" w932 {
                                tunnel: w931 -> [w954 w1271]
                                tunnel: [w953 w1270] -> w930
                                tunnel: w929 -> [w955 _]
                                tunnel: w928 -> [w952 _]
                                tunnel: w927 -> [w951 _]
                                tunnel: w926 -> [w950 _]
                                tunnel: w925 -> [w949 _]
                                tunnel: w924 -> [w948 _]
                                tunnel: w923 -> [w947 _]
                                tunnel: w922 -> [w946 _]
                                tunnel: w921 -> [w945 _]
                                tunnel: w920 -> [w944 _]
                                tunnel: w919 -> [w943 _]
                                tunnel: w918 -> [w942 _]
                                tunnel: w917 -> [w941 _]
                                tunnel: w916 -> [w940 _]
                                tunnel: w915 -> [w939 _]
                                tunnel: w914 -> [w938 _]
                                tunnel: w913 -> [w937 _]
                                tunnel: w912 -> [w936 _]
                                tunnel: w911 -> [w935 _]
                                tunnel: w910 -> [w934 _]
                                tunnel: w909 -> [w933 _]
                                frame False {
                                n151 = case shown="False" w955 {
                                tunnel: w954 -> [w976 w1269]
                                tunnel: [w975 w1268] -> w953
                                tunnel: w952 -> [w977 _]
                                tunnel: w951 -> [w974 _]
                                tunnel: w950 -> [w973 _]
                                tunnel: w949 -> [w972 _]
                                tunnel: w948 -> [w971 _]
                                tunnel: w947 -> [w970 _]
                                tunnel: w946 -> [w969 _]
                                tunnel: w945 -> [w968 _]
                                tunnel: w944 -> [w967 _]
                                tunnel: w943 -> [w966 _]
                                tunnel: w942 -> [w965 _]
                                tunnel: w941 -> [w964 _]
                                tunnel: w940 -> [w963 _]
                                tunnel: w939 -> [w962 _]
                                tunnel: w938 -> [w961 _]
                                tunnel: w937 -> [w960 _]
                                tunnel: w936 -> [w959 _]
                                tunnel: w935 -> [w958 _]
                                tunnel: w934 -> [w957 _]
                                tunnel: w933 -> [w956 _]
                                frame False {
                                n152 = case shown="False" w977 {
                                tunnel: w976 -> [w997 w1266]
                                tunnel: [w996 w1264] -> w975
                                tunnel: w974 -> [w998 _]
                                tunnel: w973 -> [w995 _]
                                tunnel: w972 -> [w994 _]
                                tunnel: w971 -> [w993 _]
                                tunnel: w970 -> [w992 _]
                                tunnel: w969 -> [w991 _]
                                tunnel: w968 -> [w990 _]
                                tunnel: w967 -> [w989 _]
                                tunnel: w966 -> [w988 _]
                                tunnel: w965 -> [w987 _]
                                tunnel: w964 -> [w986 _]
                                tunnel: w963 -> [w985 _]
                                tunnel: w962 -> [w984 _]
                                tunnel: w961 -> [w983 _]
                                tunnel: w960 -> [w982 _]
                                tunnel: w959 -> [w981 _]
                                tunnel: w958 -> [w980 _]
                                tunnel: w957 -> [w979 _]
                                tunnel: w956 -> [w978 _]
                                frame False {
                                n153 = case shown="False" w998 {
                                tunnel: w997 -> [w1017 w1262]
                                tunnel: [w1016 w1261] -> w996
                                tunnel: w995 -> [w1018 _]
                                tunnel: w994 -> [w1015 _]
                                tunnel: w993 -> [w1014 _]
                                tunnel: w992 -> [w1013 _]
                                tunnel: w991 -> [w1012 _]
                                tunnel: w990 -> [w1011 _]
                                tunnel: w989 -> [w1010 _]
                                tunnel: w988 -> [w1009 _]
                                tunnel: w987 -> [w1008 _]
                                tunnel: w986 -> [w1007 _]
                                tunnel: w985 -> [w1006 _]
                                tunnel: w984 -> [w1005 _]
                                tunnel: w983 -> [w1004 _]
                                tunnel: w982 -> [w1003 _]
                                tunnel: w981 -> [w1002 _]
                                tunnel: w980 -> [w1001 _]
                                tunnel: w979 -> [w1000 _]
                                tunnel: w978 -> [w999 _]
                                frame False {
                                n154 = case shown="False" w1018 {
                                tunnel: w1017 -> [w1036 w1259]
                                tunnel: [w1035 w1258] -> w1016
                                tunnel: w1015 -> [w1037 _]
                                tunnel: w1014 -> [w1034 _]
                                tunnel: w1013 -> [w1033 _]
                                tunnel: w1012 -> [w1032 _]
                                tunnel: w1011 -> [w1031 _]
                                tunnel: w1010 -> [w1030 _]
                                tunnel: w1009 -> [w1029 _]
                                tunnel: w1008 -> [w1028 _]
                                tunnel: w1007 -> [w1027 _]
                                tunnel: w1006 -> [w1026 _]
                                tunnel: w1005 -> [w1025 _]
                                tunnel: w1004 -> [w1024 _]
                                tunnel: w1003 -> [w1023 _]
                                tunnel: w1002 -> [w1022 _]
                                tunnel: w1001 -> [w1021 _]
                                tunnel: w1000 -> [w1020 _]
                                tunnel: w999 -> [w1019 _]
                                frame False {
                                n155 = case shown="False" w1037 {
                                tunnel: w1036 -> [w1054 w1257]
                                tunnel: [w1053 w1255] -> w1035
                                tunnel: w1034 -> [w1055 _]
                                tunnel: w1033 -> [w1052 _]
                                tunnel: w1032 -> [w1051 _]
                                tunnel: w1031 -> [w1050 _]
                                tunnel: w1030 -> [w1049 _]
                                tunnel: w1029 -> [w1048 _]
                                tunnel: w1028 -> [w1047 _]
                                tunnel: w1027 -> [w1046 _]
                                tunnel: w1026 -> [w1045 _]
                                tunnel: w1025 -> [w1044 _]
                                tunnel: w1024 -> [w1043 _]
                                tunnel: w1023 -> [w1042 _]
                                tunnel: w1022 -> [w1041 _]
                                tunnel: w1021 -> [w1040 _]
                                tunnel: w1020 -> [w1039 _]
                                tunnel: w1019 -> [w1038 _]
                                frame False {
                                n156 = case shown="False" w1055 {
                                tunnel: w1054 -> [w1071 w1253]
                                tunnel: [w1070 w1252] -> w1053
                                tunnel: w1052 -> [w1072 _]
                                tunnel: w1051 -> [w1069 _]
                                tunnel: w1050 -> [w1068 _]
                                tunnel: w1049 -> [w1067 _]
                                tunnel: w1048 -> [w1066 _]
                                tunnel: w1047 -> [w1065 _]
                                tunnel: w1046 -> [w1064 _]
                                tunnel: w1045 -> [w1063 _]
                                tunnel: w1044 -> [w1062 _]
                                tunnel: w1043 -> [w1061 _]
                                tunnel: w1042 -> [w1060 _]
                                tunnel: w1041 -> [w1059 _]
                                tunnel: w1040 -> [w1058 _]
                                tunnel: w1039 -> [w1057 _]
                                tunnel: w1038 -> [w1056 _]
                                frame False {
                                n157 = case shown="False" w1072 {
                                tunnel: w1071 -> [w1087 w1250]
                                tunnel: [w1086 w1249] -> w1070
                                tunnel: w1069 -> [w1088 _]
                                tunnel: w1068 -> [w1085 _]
                                tunnel: w1067 -> [w1084 _]
                                tunnel: w1066 -> [w1083 _]
                                tunnel: w1065 -> [w1082 _]
                                tunnel: w1064 -> [w1081 _]
                                tunnel: w1063 -> [w1080 _]
                                tunnel: w1062 -> [w1079 _]
                                tunnel: w1061 -> [w1078 _]
                                tunnel: w1060 -> [w1077 _]
                                tunnel: w1059 -> [w1076 _]
                                tunnel: w1058 -> [w1075 _]
                                tunnel: w1057 -> [w1074 _]
                                tunnel: w1056 -> [w1073 _]
                                frame False {
                                n158 = case shown="False" w1088 {
                                tunnel: w1087 -> [w1102 w1248]
                                tunnel: [w1101 w1246] -> w1086
                                tunnel: w1085 -> [w1103 _]
                                tunnel: w1084 -> [w1100 _]
                                tunnel: w1083 -> [w1099 _]
                                tunnel: w1082 -> [w1098 _]
                                tunnel: w1081 -> [w1097 _]
                                tunnel: w1080 -> [w1096 _]
                                tunnel: w1079 -> [w1095 _]
                                tunnel: w1078 -> [w1094 _]
                                tunnel: w1077 -> [w1093 _]
                                tunnel: w1076 -> [w1092 _]
                                tunnel: w1075 -> [w1091 _]
                                tunnel: w1074 -> [w1090 _]
                                tunnel: w1073 -> [w1089 _]
                                frame False {
                                n159 = case shown="False" w1103 {
                                tunnel: w1102 -> [w1116 w1245]
                                tunnel: [w1115 w1243] -> w1101
                                tunnel: w1100 -> [w1117 _]
                                tunnel: w1099 -> [w1114 _]
                                tunnel: w1098 -> [w1113 _]
                                tunnel: w1097 -> [w1112 _]
                                tunnel: w1096 -> [w1111 _]
                                tunnel: w1095 -> [w1110 _]
                                tunnel: w1094 -> [w1109 _]
                                tunnel: w1093 -> [w1108 _]
                                tunnel: w1092 -> [w1107 _]
                                tunnel: w1091 -> [w1106 _]
                                tunnel: w1090 -> [w1105 _]
                                tunnel: w1089 -> [w1104 _]
                                frame False {
                                n160 = case shown="False" w1117 {
                                tunnel: [w1129 w1242] -> w1115
                                tunnel: w1116 -> [w1128 w1240]
                                tunnel: w1114 -> [w1130 _]
                                tunnel: w1113 -> [w1127 _]
                                tunnel: w1112 -> [w1126 _]
                                tunnel: w1111 -> [w1125 _]
                                tunnel: w1110 -> [w1124 _]
                                tunnel: w1109 -> [w1123 _]
                                tunnel: w1108 -> [w1122 _]
                                tunnel: w1107 -> [w1121 _]
                                tunnel: w1106 -> [w1120 _]
                                tunnel: w1105 -> [w1119 _]
                                tunnel: w1104 -> [w1118 _]
                                frame False {
                                n161 = case shown="False" w1130 {
                                tunnel: [w1140 w1239] -> w1129
                                tunnel: w1128 -> [w1141 w1237]
                                tunnel: w1127 -> [w1142 _]
                                tunnel: w1126 -> [w1139 _]
                                tunnel: w1125 -> [w1138 _]
                                tunnel: w1124 -> [w1137 _]
                                tunnel: w1123 -> [w1136 _]
                                tunnel: w1122 -> [w1135 _]
                                tunnel: w1121 -> [w1134 _]
                                tunnel: w1120 -> [w1133 _]
                                tunnel: w1119 -> [w1132 _]
                                tunnel: w1118 -> [w1131 _]
                                frame False {
                                n162 = case shown="False" w1142 {
                                tunnel: w1141 -> [w1152 w1235]
                                tunnel: [w1151 w1234] -> w1140
                                tunnel: w1139 -> [w1153 _]
                                tunnel: w1138 -> [w1150 _]
                                tunnel: w1137 -> [w1149 _]
                                tunnel: w1136 -> [w1148 _]
                                tunnel: w1135 -> [w1147 _]
                                tunnel: w1134 -> [w1146 _]
                                tunnel: w1133 -> [w1145 _]
                                tunnel: w1132 -> [w1144 _]
                                tunnel: w1131 -> [w1143 _]
                                frame False {
                                n163 = case shown="False" w1153 {
                                tunnel: w1152 -> [w1162 w1233]
                                tunnel: [w1161 w1231] -> w1151
                                tunnel: w1150 -> [w1163 _]
                                tunnel: w1149 -> [w1160 _]
                                tunnel: w1148 -> [w1159 _]
                                tunnel: w1147 -> [w1158 _]
                                tunnel: w1146 -> [w1157 _]
                                tunnel: w1145 -> [w1156 _]
                                tunnel: w1144 -> [w1155 _]
                                tunnel: w1143 -> [w1154 _]
                                frame False {
                                n164 = case shown="False" w1163 {
                                tunnel: w1162 -> [w1171 w1230]
                                tunnel: [w1170 w1228] -> w1161
                                tunnel: w1160 -> [w1172 _]
                                tunnel: w1159 -> [w1169 _]
                                tunnel: w1158 -> [w1168 _]
                                tunnel: w1157 -> [w1167 _]
                                tunnel: w1156 -> [w1166 _]
                                tunnel: w1155 -> [w1165 _]
                                tunnel: w1154 -> [w1164 _]
                                frame False {
                                n165 = case shown="False" w1172 {
                                tunnel: w1171 -> [w1179 w1227]
                                tunnel: [w1178 w1225] -> w1170
                                tunnel: w1169 -> [w1180 _]
                                tunnel: w1168 -> [w1177 _]
                                tunnel: w1167 -> [w1176 _]
                                tunnel: w1166 -> [w1175 _]
                                tunnel: w1165 -> [w1174 _]
                                tunnel: w1164 -> [w1173 _]
                                frame False {
                                n166 = case shown="False" w1180 {
                                tunnel: w1179 -> [w1186 w1223]
                                tunnel: [w1185 w1222] -> w1178
                                tunnel: w1177 -> [w1187 _]
                                tunnel: w1176 -> [w1184 _]
                                tunnel: w1175 -> [w1183 _]
                                tunnel: w1174 -> [w1182 _]
                                tunnel: w1173 -> [w1181 _]
                                frame False {
                                n167 = case shown="False" w1187 {
                                tunnel: w1186 -> [w1192 w1220]
                                tunnel: [w1191 w1219] -> w1185
                                tunnel: w1184 -> [w1193 _]
                                tunnel: w1183 -> [w1190 _]
                                tunnel: w1182 -> [w1189 _]
                                tunnel: w1181 -> [w1188 _]
                                frame False {
                                n168 = case shown="False" w1193 {
                                tunnel: w1192 -> [w1197 w1218]
                                tunnel: [w1196 w1217] -> w1191
                                tunnel: w1190 -> [w1198 _]
                                tunnel: w1189 -> [w1195 _]
                                tunnel: w1188 -> [w1194 _]
                                frame False {
                                n169 = case shown="False" w1198 {
                                tunnel: w1197 -> [w1201 w1215]
                                tunnel: [w1200 w1214] -> w1196
                                tunnel: w1195 -> [w1202 _]
                                tunnel: w1194 -> [w1199 _]
                                frame False {
                                n170 = case shown="False" w1202 {
                                tunnel: w1201 -> [w1203 w1212]
                                tunnel: [w1204 w1211] -> w1200
                                tunnel: w1199 -> [w1205 _]
                                frame False {
                                n171 = case shown="False" w1205 {
                                tunnel: w1203 -> [_ w1209]
                                tunnel: [w1206 w1208] -> w1204
                                tunnel: w1203 -> [w1206 _]
                                frame False {
                                }
                                frame True {
                                n172 = Multiply(x=w1209, y=5280) -> (x*y=w1208:dbl)
                                }
                                }
                                }
                                frame True {
                                n173 = Divide(x=w1212, y=5280) -> (x/y=w1211:dbl)
                                }
                                }
                                }
                                frame True {
                                n174 = Multiply(x=w1215, y=63360) -> (x*y=w1214:dbl)
                                }
                                }
                                }
                                frame True {
                                n175 = Divide(x=w1218, y=63360) -> (x/y=w1217:dbl)
                                }
                                }
                                }
                                frame True {
                                n176 = Multiply(x=w1220, y=12) -> (x*y=w1219:dbl)
                                }
                                }
                                }
                                frame True {
                                n177 = Divide(x=w1223, y=12) -> (x/y=w1222:dbl)
                                }
                                }
                                }
                                frame True {
                                n178 = Multiply(x=w1227, y=1.609) -> (x*y=w1225:dbl)
                                }
                                }
                                }
                                frame True {
                                n179 = Divide(x=w1230, y=1.609) -> (x/y=w1228:dbl)
                                }
                                }
                                }
                                frame True {
                                n180 = Divide(x=w1233, y=3281) -> (x/y=w1231:dbl)
                                }
                                }
                                }
                                frame True {
                                n181 = Multiply(x=w1235, y=3281) -> (x*y=w1234:dbl)
                                }
                                }
                                }
                                frame True {
                                n182 = Divide(x=w1237, y=39370) -> (x/y=w1239:dbl)
                                }
                                }
                                }
                                frame True {
                                n183 = Multiply(x=w1240, y=39370) -> (x*y=w1242:dbl)
                                }
                                }
                                }
                                frame True {
                                n184 = Multiply(x=w1245, y=1609) -> (x*y=w1243:dbl)
                                }
                                }
                                }
                                frame True {
                                n185 = Divide(x=w1248, y=1609) -> (x/y=w1246:dbl)
                                }
                                }
                                }
                                frame True {
                                n186 = Divide(x=w1250, y=3.281) -> (x/y=w1249:dbl)
                                }
                                }
                                }
                                frame True {
                                n187 = Multiply(x=w1253, y=3.281) -> (x*y=w1252:dbl)
                                }
                                }
                                }
                                frame True {
                                n188 = Divide(x=w1257, y=39.37) -> (x/y=w1255:dbl)
                                }
                                }
                                }
                                frame True {
                                n189 = Multiply(x=w1259, y=39.37) -> (x*y=w1258:dbl)
                                }
                                }
                                }
                                frame True {
                                n190 = Multiply(x=w1262, y=1000) -> (x*y=w1261:dbl)
                                }
                                }
                                }
                                frame True {
                                n191 = Divide(x=w1266, y=1000) -> (x/y=w1264:dbl)
                                }
                                }
                                }
                                frame True {
                                n192 = Multiply(x=w1269, y=160934) -> (x*y=w1268:dbl)
                                }
                                }
                                }
                                frame True {
                                n193 = Divide(x=w1271, y=0) -> (x/y=w1270:dbl)
                                }
                                }
                                }
                                frame True {
                                n194 = Multiply(x=w1275, y=30.48) -> (x*y=w1273:dbl)
                                }
                                }
                                }
                                frame True {
                                n195 = Divide(x=w1277, y=30.48) -> (x/y=w1276:dbl)
                                }
                                }
                                }
                                frame True {
                                n196 = Multiply(x=w1281, y=2.54) -> (x*y=w1279:dbl)
                                }
                                }
                                }
                                frame True {
                                n197 = Divide(x=w1283, y=2.54) -> (x/y=w1282:dbl)
                                }
                                }
                                }
                                frame True {
                                n198 = Multiply(x=w1287, y=100000) -> (x*y=w1285:dbl)
                                }
                                }
                                }
                                frame True {
                                n199 = Divide(x=w1289, y=100000) -> (x/y=w1288:dbl)
                                }
                                }
                                }
                                frame True {
                                n200 = Multiply(x=w1293, y=100) -> (x*y=w1291:dbl)
                                }
                                }
                                }
                                frame True {
                                n201 = Divide(x=w1295, y=100) -> (x/y=w1294:dbl)
                                }
                                }
                                }
                                frame True {
                                n202 = Multiply(x=w1298, y=1609344) -> (x*y=w1297:dbl)
                                }
                                }
                                }
                                frame True {
                                n203 = Divide(x=w1301, y=1609344) -> (x/y=w1300:dbl)
                                }
                                }
                                }
                                frame True {
                                n204 = Multiply(x=w1305, y=305) -> (x*y=w1303:dbl)
                                }
                                }
                                }
                                frame True {
                                n205 = Divide(x=w1307, y=305) -> (x/y=w1306:dbl)
                                }
                                }
                                }
                                frame True {
                                n206 = Multiply(x=w1311, y=25.4) -> (x*y=w1309:dbl)
                                }
                                }
                                }
                                frame True {
                                n207 = Divide(x=w1314, y=25.4) -> (x/y=w1312:dbl)
                                }
                                }
                              }
                              frame True {
                                n208 = Multiply(x=w1316, y=1000000) -> (x*y=w1315:dbl)
                              }
                            }
                          }
                          frame True {
                            n209 = Divide(x=w1319, y=1000000) -> (x/y=w1318:dbl)
                          }
                        }
                      }
                      frame True {
                        n210 = Multiply(x=w1323, y=1000) -> (x*y=w1321:dbl)
                      }
                    }
                  }
                  frame True {
                    n211 = Divide(x=w1326, y=1000) -> (x/y=w1324:dbl)
                  }
                }
              }
              frame True {
                n212 = Multiply(x=w1329, y=10) -> (x*y=w1327:dbl)
              }
            }
          }
          frame True {
            n213 = Divide(x=w1332, y=10) -> (x/y=w1330:dbl)
          }
        }
      }
    }
    "Value of destiny scale" <- w210
  }
